vi "Client.vi"() -> ()   [LabVIEW 2013, in "OPC UA Demo.lvlib"]
doc: "Demonstrates the use of the <B>OPC UA Client VIs</B> to programmatically create an OPC UA client and connects the OPC UA client to an OPC UA server."
uses:
  OPC UA Demo.lvlib
  <vilib>/OPCUA/client/Write Int32.vi
  <vilib>/OPCUA/NI OPC UA Client.lvlib
  <vilib>/OPCUA/NI OPC UA Utility.lvlib
panel:
  in  "security policy":T1={"message mode"=enum."Sign", "security"=enum."Basic256"}
  in  "Device.Node.Set Point":i32=1000
  out "error out":errorcluster
  out "Waveform Chart":i32(graph)
  in  "stop":bool
  in  "server endpoint URL":string="opc.tcp://localhost:49580"
  # "Overview: Demonstrates the use of the OPC UA Client VIs to programmatically create an OPC UA client and connects the OPC UA client to an OPC UA server.\nRequirements: \n1. LabVIEW Datalogging and Supervisory Control Module or LabVIEW Real-Time Module\n2. (Real-Time Module) RT target\nInstructions:\nRun the VI."
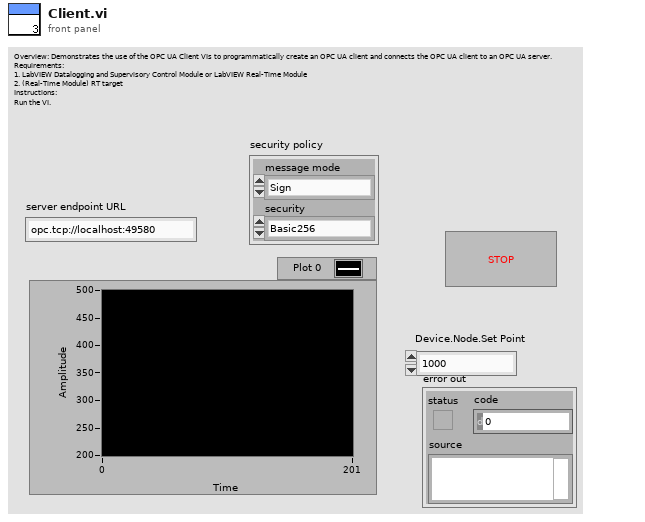
[diagram p1: front panel]
types:
  T1 = cluster{"message mode":enum16{"None", "Sign", "Sign and Encrypt"}, "security":enum16{"Basic256", "Basic128Rsa15"}}
  T2 = cluster{"Item URL":string, "Item Value":variant, "Timestamp":timestamp, "DataType":u32, "status code":u32}[]
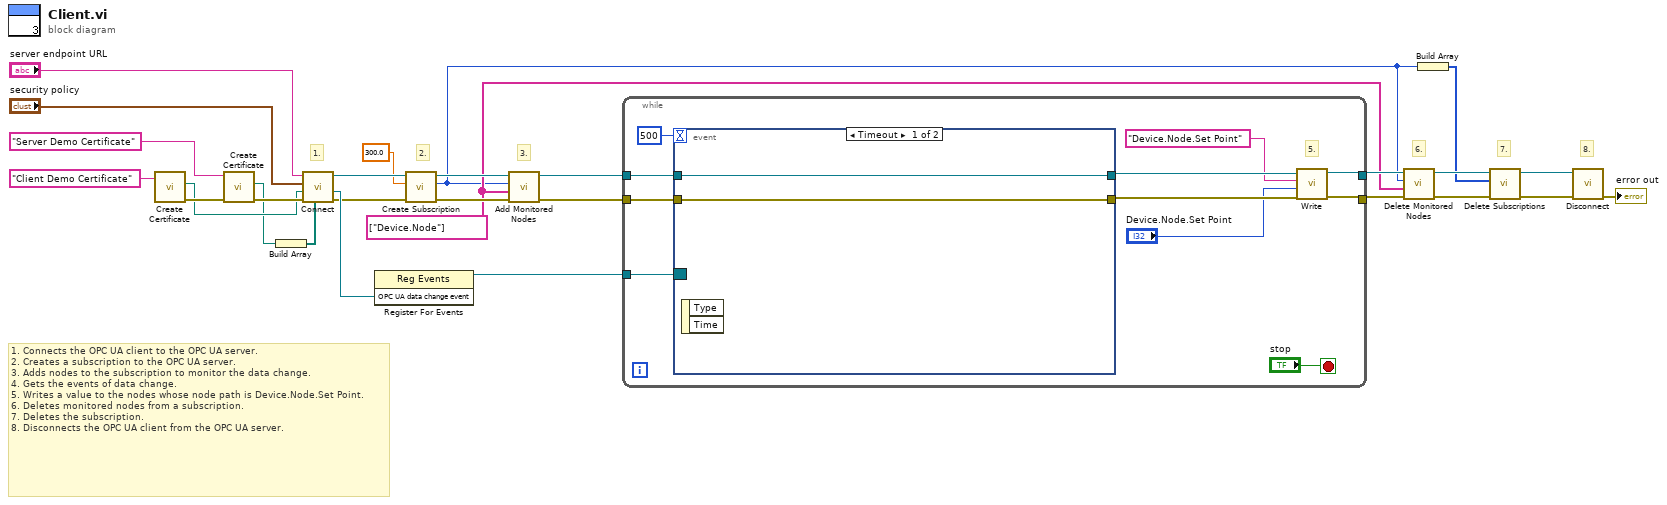
[diagram p0: block diagram]
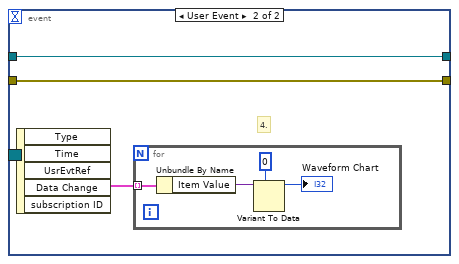
[diagram p2: hidden frame]
diagram:
  w12 = string[] ["Device.Node"] ("array of node path")
  # "7."
  # "1. Connects the OPC UA client to the OPC UA server. \n2. Creates a subscription to the OPC UA server.\n3. Adds nodes to the subscription to monitor the data change.\n4. Gets the events of data change.\n5. Writes a value to the nodes whose node path is Device.Node.Set Point. \n6. Deletes monitored nodes from a subscription.\n7. Deletes the subscription.\n8. Disconnects the OPC UA client from the OPC UA server."
  # "8."
  # "6."
  # "3."
  # "2."
  # "1."
  n1 = call <vilib>:"Create Certificate.vi"("certificate name in"="Client Demo Certificate") -> ("error out"=w7:errorcluster, "certificate path"=w2:path)  [unwired: 7 in, 2 out]
  n2 = call <vilib>:"Create Certificate.vi"("error in (no error)"=w7, "certificate name in"="Server Demo Certificate") -> ("error out"=w6:errorcluster, "certificate path"=w1:path)  [unwired: 6 in, 2 out]
  n3 = Build Array(w1) -> (w4:path[])
  n4 = call <vilib>:"Connect.vi"("trusted server certificates"=w4, "error in (no error)"=w6, "client certificate file"=w2, "security policy"="security policy", "server endpoint URL"="server endpoint URL") -> ("error out"=w14:errorcluster, "OPC UA data change event"=w25:refnum<user-event>, "OPC UA client refnum out"=w15:refnum<k21>)  [unwired: 4 in]
  n5 = register-events(w25) -> (reference out=w24:refnum<event-registration>)  [unwired: 2 in, 1 out]
  n6 = call <vilib>:"Create Subscription.vi"("error in (no error)"=w14, "update rate (1000 ms)"=300.0, "OPC UA client refnum in"=w15) -> ("error out"=w26:errorcluster, "subscription ID out"=w11:u32, "OPC UA client refnum out"=w27:refnum<k21>)  [unwired: 6 in]
  n7 = call <vilib>:"Add Monitored Nodes.vi"("error in (no error)"=w26, "array of node path"=w12, "subscription ID in"=w11, "OPC UA client refnum in"=w27) -> ("error out"=w22:errorcluster, "OPC UA client refnum out"=w23:refnum<k21>)  [unwired: 5 in, 1 out]
  n8 = while {
    tunnel: w24 -> [w39]
    tunnel: w23 -> [w37]
    tunnel: w22 -> [w36]
    tunnel: [w32] -> w20
    tunnel: [w34] -> w21
    stop <- "stop" stop-if-true
    # "5."
    n9 = event shown="[0] Timeout" {
      selector: w39 -> [_ _]
      dyn-events: _ -> [_ _]
      timeout: 500 -> [_ _]
      tunnel: w37 -> [w41 w44]
      tunnel: w36 -> [w40 w43]
      tunnel: [w41 w44] -> w35
      tunnel: [w40 w43] -> w33
      event Timeout {
        n10 = event-data() -> ()  [unwired: 1 in, 2 out]
      }
      event User Event {
        # "4."
        n11 = event-data() -> ("Data Change"=w42:T2)  [unwired: 1 in, 4 out]
        n12 = for {
          tunnel: w42 -> [w48] mode=indexing
          n13 = Unbundle By Name(w48) -> ("Item Value"=w47:variant)
          n14 = Variant To Data(type=0, Variant=w47) -> (data=→"Waveform Chart":i32)  [unwired: 1 in, 1 out]
        }
      }
    }
    n15 = call-poly <vilib>:"Write.vi"("error in (no error)"=w33, "value"="Device.Node.Set Point", "node path"="Device.Node.Set Point", "OPC UA client refnum in"=w35) -> ("error out"=w32:errorcluster, "OPC UA client refnum out"=w34:refnum<k21>)  [unwired: 5 in, 1 out]
  }
  n16 = call <vilib>:"Delete Monitored Nodes.vi"("error in (no error)"=w20, "array of node path"=w12, "subscription ID in"=w11, "OPC UA client refnum in"=w21) -> ("error out"=w18:errorcluster, "OPC UA client refnum out"=w19:refnum<k21>)  [unwired: 4 in, 2 out]
  n17 = Build Array(w11) -> (w10:u32[])
  n18 = call <vilib>:"Delete Subscriptions.vi"("error in (no error)"=w18, "array of subscription ID"=w10, "OPC UA client refnum in"=w19) -> ("error out"=w16:errorcluster, "OPC UA client refnum out"=w17:refnum<k21>)  [unwired: 6 in, 1 out]
  n19 = call <vilib>:"Disconnect.vi"("error in (no error)"=w16, "OPC UA client refnum in"=w17) -> ("error out"=→"error out":errorcluster)  [unwired: 9 in]
